vi "Sweep Voltage.vi"() -> ()   [LabVIEW 2017, in "LCD Retarder.lvclass"]
uses:
  LCD Retarder.lvclass
  DAQ/DAQmx Analog.lvclass
  C:/LabVIEW-programs-dev/Instruments/Utility Classes/Readable/Readable.lvclass
  <vilib>/Analysis/baseanly.llb/Mean (DBL).vi
  Utility Classes/Readable/Readable.lvclass
  <vilib>/Analysis/NI_AALBase.lvlib
panel:
  out "Smoothed Graph":cluster{"Y":dbl[], "Y":dbl[]}[](graph)
  out "Run #":dbl
  in  "Averages":dbl
  out "Current Retardance":dbl[unit]
  out "?":dbl
  out "Minimum":dbl
  in  "Analog DAQ Ch#":i32
  in  "Ending Voltage":dbl
  in  "Starting Voltage":dbl
  out "LCD curve":cluster{"Y":dbl[], "Y":dbl[]}[](graph)
  # "at LCD Voltage"
  # "V"
  # "Volts"
  # "Volts"
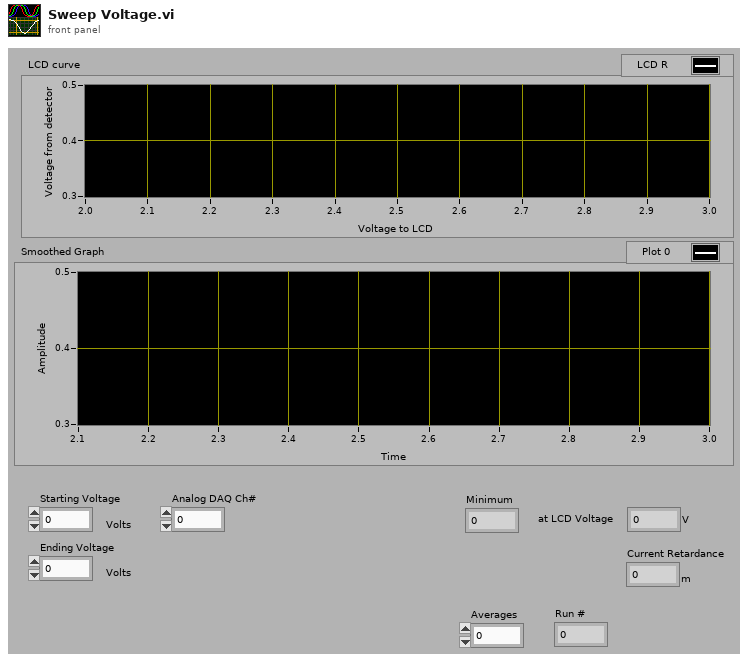
[diagram p1: front panel]
types:
  T1 = typedef "Readable.lvclass/X array.ctl" = T2[]
  T2 = typedef "Readable.lvclass/X.ctl" = dbl
  T3 = cluster{"Channel Names[0]":string, "Channel Names[1]":string, "Channel Names[2]":string, "Channel Names[3]":string, "Channel Names[4]":string, "Channel Names[5]":string, "Channel Names[6]":string, "Channel Names[7]":string, "Channel Names[8]":string}
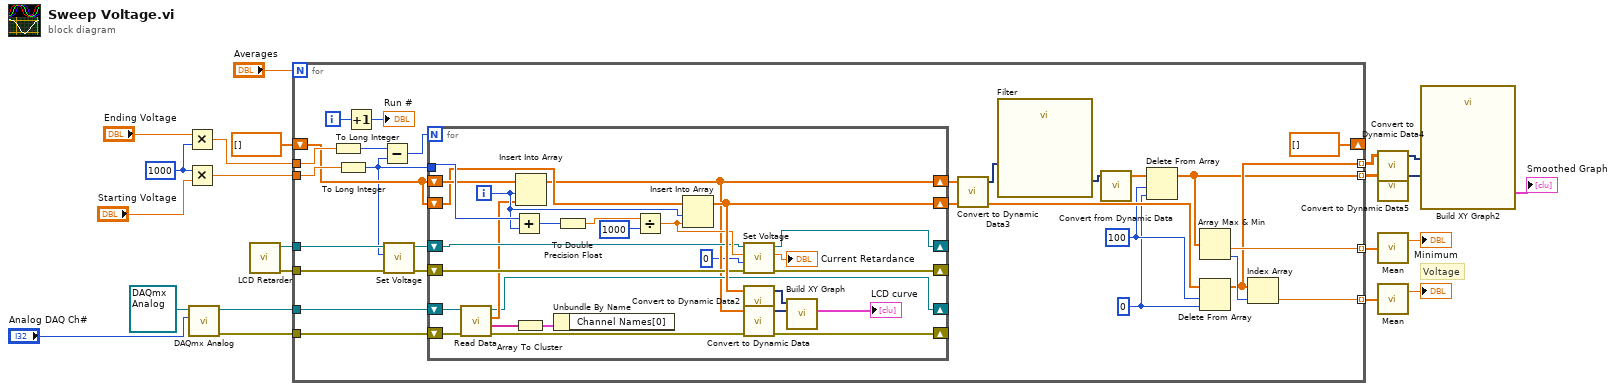
[diagram p0: block diagram]
diagram:
  w22 = 1000
  # "Voltage"
  n1 = Multiply(x="Ending Voltage", y=w22) -> (x*y=w20:dbl)
  n2 = Multiply(x=w22, y="Starting Voltage") -> (x*y=w21:dbl)
  n3 = call "DAQmx Analog.vi"("Analog input #"="Analog DAQ Ch#", "DAQmx Analog in"=refnum<class "DAQmx Analog.lvclass"> refnum ("DAQmx Analog.lvclass")) -> ("error out"=w12:errorcluster, "DAQmx Analog out"=w13:refnum<class "DAQmx Analog.lvclass">)  [unwired: 8 in]
  n4 = call "LCD Retarder.vi"() -> ("errorOUT"=w14:errorcluster, "LCD out"=w15:refnum<class "LCD Retarder.lvclass">)  [unwired: 10 in]
  n5 = for {
    N: "Averages" -> [_]
    tunnel: w21 -> [w49]
    tunnel: w20 -> [w47]
    tunnel: w15 -> [w27]
    tunnel: w14 -> [w24]
    tunnel: w13 -> [w44]
    tunnel: w12 -> [w43]
    shift-right: [dbl[] []] -> _
    shift-left: dbl[] [] -> [w46]
    tunnel: [w42] -> w9 mode=indexing
    tunnel: [w30] -> w3 mode=indexing
    tunnel: [w29] -> w2 mode=indexing
    tunnel: [w28] -> w1 mode=indexing
    i -> [w40]
    w33 = 100
    w32 = 0
    n6 = To Long Integer(number=w47) -> (32bit integer=w48:i32)
    n7 = To Long Integer(number=w49) -> (32bit integer=w25:i32)
    n8 = Increment(x=w40) -> (x+1=→"Run #":i32)
    n9 = Subtract(x=w48, y=w25) -> (x-y=w45:i32)
    n10 = call "Set Voltage.vi"("errorIN"=w24, "Voltage in"=w25, "LCD in"=w27) -> ("errorOUT"=w23:errorcluster, "LCD out"=w26:refnum<class "LCD Retarder.lvclass">)  [unwired: 6 in, 1 out]
    n11 = for {
      N: w45 -> [_]
      shift-right: [w54] -> _
      shift-left: w44 -> [w63]
      shift-right: [w60] -> _
      shift-left: w23 -> [w66]
      shift-right: [w59] -> _
      shift-left: w26 -> [w64]
      shift-right: [w53] -> _
      shift-left: w43 -> [w62]
      tunnel: w25 -> [w71]
      shift-right: [w51] -> w38
      shift-left: w46 -> [w70]
      shift-right: [w67] -> w36
      shift-left: w46 -> [w69]
      i -> [w68]
      n12 = call "Read Data.vi"("error in (no error)"=w62, "Readable in"=w63) -> ("error out"=w53:errorcluster, "Channel Names"=w61:string[], "X array"=w55:T1, "Readable out"=w54:refnum<class "DAQmx Analog.lvclass">)  [unwired: 3 in, 3 out]
      n13 = Add(x=w71, y=w68) -> (x+y=w72:i32)
      n14 = Array To Cluster(array=w61) -> (cluster=w75:T3)
      n15 = Insert Into Array(array=w70, index=w68, new element=w55) -> (w51:dbl[])
      n16 = Unbundle By Name(w75) -> ()  [unwired: 1 out]
      n17 = To Double Precision Float(number=w72) -> (double precision float=w74:dbl)
      n18 = Divide(x=w74, y=1000) -> (x/y=w65:dbl)
      n19 = Insert Into Array(array=w69, index=w68, new element=w65) -> (w67:dbl[])
      n20 = call "Set Voltage.vi"("errorIN"=w66, "milliseconds to wait (0)"=0, "Voltage in"=w65, "LCD in"=w64) -> ("errorOUT"=w60:errorcluster, "Retardance out"=→"Current Retardance":dbl[unit], "LCD out"=w59:refnum<class "LCD Retarder.lvclass">)  [unwired: 5 in]
      n21 = call "Convert to Dynamic Data2"("Array"=w67) -> ("Dynamic Data Type"=w58:dynamicdata)  [unwired: 3 in]
      n22 = call "Convert to Dynamic Data"("Array"=w51) -> ("Dynamic Data Type"=w57:dynamicdata)  [unwired: 3 in]
      n23 = call "Build XY Graph"("Y Input"=w57, "X Input"=w58) -> ("XY Graph"=→"LCD curve":cluster{"Y":dbl[], "Y":dbl[]}[])  [unwired: 8 in, 1 out]
    }
    n24 = call "Convert to Dynamic Data3"("Array"=w38) -> ("Dynamic Data Type"=w37:dynamicdata)  [unwired: 3 in]
    n25 = call "Filter"("Signal"=w37) -> ("Filtered Signal"=w35:dynamicdata)  [unwired: 9 in, 1 out]
    n26 = call "Convert from Dynamic Data"("Dynamic Data Type"=w35) -> ("Array"=w34:dbl[])  [unwired: 3 in]
    n27 = Delete From Array(array=w34, length=w33, index=w32) -> (array with subset deleted=w28:dbl[])  [unwired: 1 out]
    n28 = Array Max & Min(array=w28) -> (min value=w42:dbl, min index (indices)=w31:i32)  [unwired: 2 out]
    n29 = Delete From Array(array=w36, length=w33, index=w32) -> (array with subset deleted=w29:dbl[])  [unwired: 1 out]
    n30 = Index Array(array=w29, index=w31) -> (element=w30:dbl)
  }
  n31 = call "Convert to Dynamic Data4"("2D Array"=w2) -> ("Dynamic Data Type"=w5:dynamicdata)  [unwired: 3 in]
  n32 = call "Convert to Dynamic Data5"("2D Array"=w1) -> ("Dynamic Data Type"=w4:dynamicdata)  [unwired: 3 in]
  n33 = call-poly <vilib>:"Mean.vi"("X"=w9) -> ("mean"=→"Minimum":dbl)  [unwired: 1 out]
  n34 = call-poly <vilib>:"Mean.vi"("X"=w3) -> ("mean"=→"?":dbl)  [unwired: 1 out]
  n35 = call "Build XY Graph2"("Y Input"=w4, "X Input"=w5) -> ("XY Graph"=→"Smoothed Graph":cluster{"Y":dbl[], "Y":dbl[]}[])  [unwired: 8 in, 1 out]
